vi "SquareWaveGenerator.vi"() -> ()   [LabVIEW 2014]
uses:
  <vilib>/MakerHub/LINX/Public/Peripherals/Digital/Digital Write 1 Chan.vi
  <vilib>/MakerHub/LINX/Public/Peripherals/Digital/Digital Write N Chans.vi
  <vilib>/MakerHub/LINX/Private/Local IO/LinxDigitalWrite.vi
  <vilib>/MakerHub/LINX/Public/Utilities/Check Channel.vi
  <vilib>/MakerHub/LINX/Private/Local IO/Handle Errors.vi
  <vilib>/MakerHub/LINX/Public/Utilities/Open Local.vi
  <vilib>/MakerHub/LINX/Private/Utilties/Generate Error.vi
  <vilib>/MakerHub/LINX/LMH-LINX.lvlib
panel:
  in  "Array":dbl[][](array[numeric])
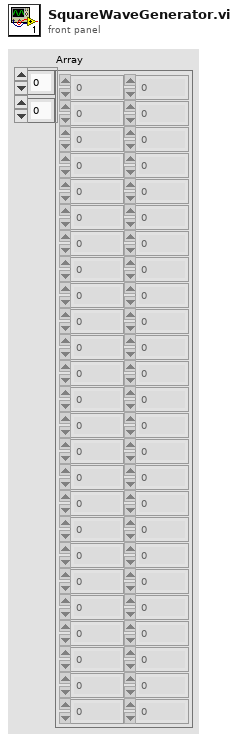
[diagram p1: front panel]
types:
  T1 = typedef "LMH-LINX.lvlib/LINX Ref.ctl" = cluster{"IO":T2, "Interface":T3, "LINX Device Config":T4}
  T2 = typedef "LMH-LINX.lvlib/Platform.ctl" = enum16{"Remote", "Local"}
  T3 = typedef "LMH-LINX.lvlib/Interface.ctl" = enum16{"Serial", "TCP"}
  T4 = typedef "LMH-LINX.lvlib/Device.lvlib/LINX Device Config.ctl" = cluster{"Interface":T3, "COM Port":refnum<visa-resource-name>, "TCP Configuration":T5, "Device Family":u8, "Device ID":u8, "Device Name":string, "TCP Ref":refnum<k5>, "Channels":T6}
  T5 = typedef "LMH-LINX.lvlib/Device.lvlib/TCP Config.ctl" = cluster{"IP Address":string, "Port":u16}
  T6 = typedef "LMH-LINX.lvlib/Channels.ctl" = cluster{"DI":u8[], "DO":u8[], "AI":u8[], "AO":u8[], "PWM":u8[], "QE":u8[], "UART":u8[], "I2C 2":u8[], "SPI":u8[], "CAN":u8[], "Servo":u8[], "AI Ref (V)":dbl, "AI Resolution (Bits)":u8, "AO Ref (V)":dbl, "AO Resolution (Bits)":u8}
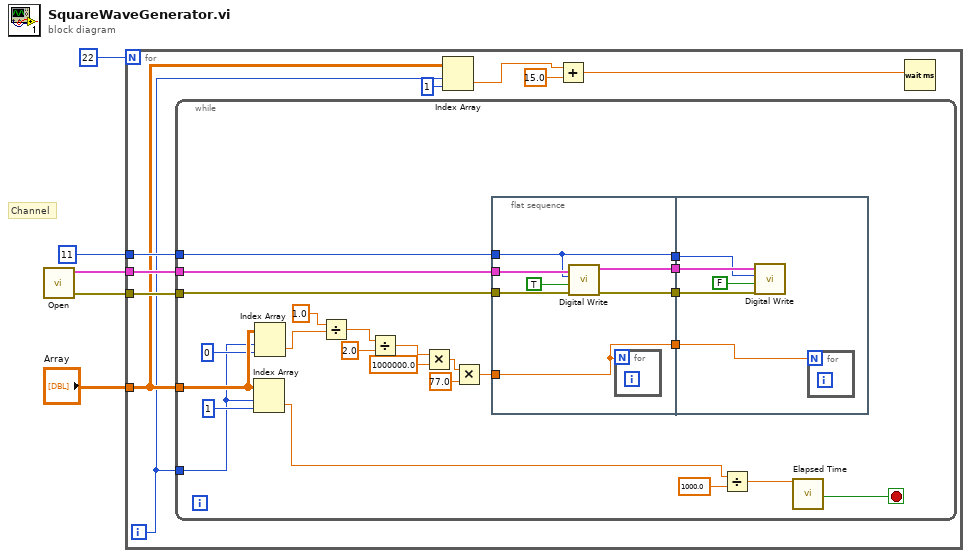
[diagram p0: block diagram]
diagram:
  # "Channel"
  n1 = call-poly <vilib>:"Open.vi"() -> ("Error Out"=w4:errorcluster, "LINX Resource"=w5:T1)  [unwired: 9 in, 1 out]
  n2 = for {
    N: 22 -> [_]
    tunnel: w5 -> [w14]
    tunnel: w4 -> [w13]
    tunnel: "Array" -> [w11]
    tunnel: 11 -> [w12]
    i -> [w10]
    n3 = while {
      tunnel: w14 -> [w35]
      tunnel: w13 -> [w34]
      tunnel: w11 -> [w22]
      tunnel: w10 -> [w16]
      tunnel: w12 -> [w15]
      stop <- w25 stop-if-true
      n4 = Index Array(array=w22, index (row)=w16, index (col)=1 ("disabled index (col)")) -> (element=w19:dbl)
      n5 = Index Array(array=w22, index (row)=w16, index (col)=0 ("disabled index (col)")) -> (element=w17:dbl)
      n6 = Divide(x=1.0, y=w17) -> (x/y=w30:dbl)
      n7 = Divide(x=w30, y=2.0) -> (x/y=w29:dbl)
      n8 = Multiply(x=w29, y=1000000.0) -> (x*y=w26:dbl)
      n9 = Multiply(x=w26, y=77.0) -> (x*y=w18:dbl)
      n10 = flat-sequence {
        tunnel: w35 -> [w44]
        tunnel: [w43] -> w38
        tunnel: w15 -> [w42]
        tunnel: [w42] -> w37
        tunnel: w34 -> [w41]
        tunnel: [w40] -> w36
        tunnel: [w39] -> w33
        tunnel: w18 -> [w39]
        tunnel: w38 -> [w49]
        tunnel: w37 -> [w48]
        tunnel: w36 -> [w47]
        tunnel: w33 -> [w46]
        frame #0 {
          n11 = call-poly <vilib>:"Digital Write.vi"("Error In"=w41, "Output Value"=TRUE, "DO Channel"=w42, "LINX Resource"=w44) -> ("Error Out"=w40:errorcluster, "LINX Resource"=w43:T1)  [unwired: 6 in]
          n12 = for {
            N: w39 -> [_]
          }
        }
        frame #1 {
          n13 = call-poly <vilib>:"Digital Write.vi"("Error In"=w47, "Output Value"=FALSE, "DO Channel"=w48, "LINX Resource"=w49) -> ()  [unwired: 6 in, 2 out]
          n14 = for {
            N: w46 -> [_]
          }
        }
      }
      n15 = Divide(x=w19, y=1000.0) -> (x/y=w23:dbl)
      n16 = call "Elapsed Time"("Time Target (s)"=w23) -> ("Time has Elapsed"=w25:bool)  [unwired: 11 in, 7 out]
    }
    n17 = Index Array(array=w11, index (row)=w10, index (col)=1 ("disabled index (col)")) -> (element=w7:dbl)
    n18 = Add(x=w7, y=15.0) -> (x+y=w6:dbl)
    n19 = Wait (ms)(milliseconds to wait=w6) -> ()  [unwired: 1 out]
  }
